vi "select data.vi"(8 "all channels":T1={"voltage data"=[0.0, 0.0, 0.0, 0.0, 0.0, 0.0048828125, 0.0, 0.0, 0.0, 0.0, 0.0024414062, 0.0024414062, 0.0, 0.0, 0.0, 0.0024414062, 0.0, 0.0048828125, 0.0024414062, 0.0048828125, 0.0, 0.0024414062, 0.0024414062, 0.0048828125, 0.01953125, 0.017089844, 0.012207031, 0.0146484375, 0.0146484375, 0.0146484375, 0.01953125, 0.009765625], "scan backlog"=0, "seconds since 1904"=0.0, "arbitrary scans"=0} {"seconds since 1904" format="%.2f"; "voltage data" format="%.4f"}, 11 "command cluster":T2={"command"=enum."Idle", "start time (ms)"=0, "Channel Indices"=[], "Scans per Sample"=1} {"Scans per Sample" min=1}) -> (0 "selected channels":T1={"voltage data"=[0.0, 0.0, 0.0, 0.0, 0.0, 0.0048828125, 0.0, 0.0, 0.0, 0.0, 0.0024414062, 0.0024414062, 0.0, 0.0, 0.0, 0.0024414062, 0.0, 0.0048828125, 0.0024414062, 0.0048828125, 0.0, 0.0024414062, 0.0024414062, 0.0048828125, 0.01953125, 0.017089844, 0.012207031, 0.0146484375, 0.0146484375, 0.0146484375, 0.01953125, 0.009765625], "scan backlog"=0, "seconds since 1904"=0.0, "arbitrary scans"=0} {"seconds since 1904" format="%.2f"; "voltage data" format="%.4f"})   [LabVIEW 2012]
uses:
  data send.ctl
  command cluster.ctl
  command.ctl
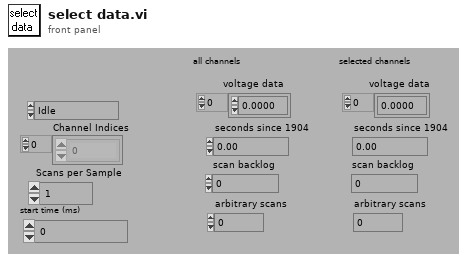
[diagram p1: front panel]
types:
  T1 = typedef "data send.ctl" = cluster{"voltage data":sgl[], "scan backlog":u32, "seconds since 1904":dbl, "arbitrary scans":i32}
  T2 = typedef "command cluster.ctl" = cluster{"command":T3, "start time (ms)":u32, "Channel Indices":i32[], "Scans per Sample":i32}
  T3 = typedef "command.ctl" = enum16{"Idle", "Send Data", "Send 1 Scan", "Logoff"}
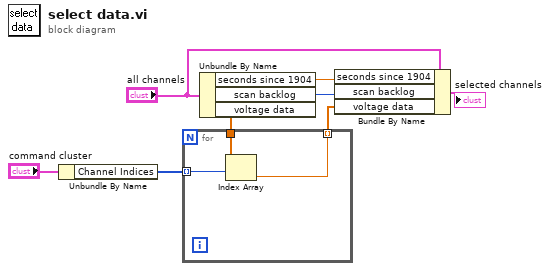
[diagram p0: block diagram]
diagram:
  n1 = Unbundle By Name("command cluster") -> ("Channel Indices"=w2:i32[])
  n2 = Unbundle By Name("all channels") -> ("seconds since 1904"=w5:dbl, "scan backlog"=w4:u32, "voltage data"=w3:sgl[])
  n3 = for {
    tunnel: w3 -> [w11]
    tunnel: w2 -> [w10] mode=indexing
    tunnel: [w9] -> w1 mode=indexing
    n4 = Index Array(array=w11, index=w10) -> (element=w9:sgl)
  }
  n5 = Bundle By Name(cluster="all channels", "seconds since 1904"=w5, "scan backlog"=w4, "voltage data"=w1) -> (→"selected channels":T1)
